vi "Update Plugin Metadata by Reference.vi"(8 "error in (no error)":errorcluster, 10 "plugin_metadata":T1, 11 "Metadata":refnum<vi>) -> (0 "error out":errorcluster)   [LabVIEW 2021, in "CIF_UI.lvclass"]
uses:
  CIF_UI.lvclass
  CIF_UI.lvclass/CIF_UI.ctl
  CIFPluginManager/CIFPluginManager/gRPC/CIF_Manager_client/RPC Messages/cif_manager_PluginMetadata.ctl
  CIFPluginManager/CIFPluginManager/gRPC/CIF_Manager_client/CIF_Manager_client.lvlib
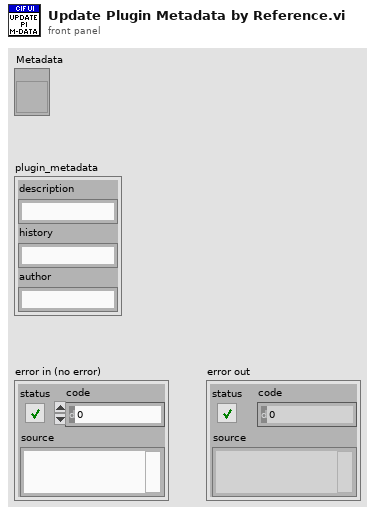
[diagram p1: front panel]
types:
  T1 = typedef "CIF_Manager_client.lvlib/cif_manager_PluginMetadata.ctl" = cluster{"description":string, "history":string, "author":string}
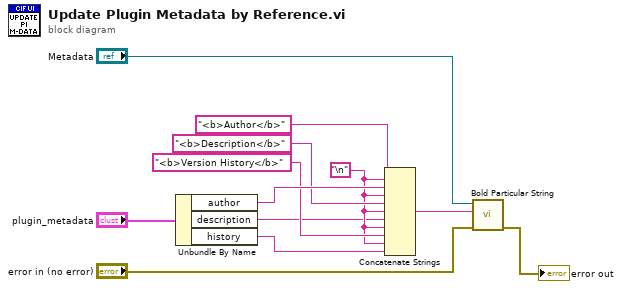
[diagram p0: block diagram]
diagram:
  w7 = "\n"
  n1 = Unbundle By Name("plugin_metadata") -> ("author"=w10:string, "description"=w6:string, "history"=w5:string)
  n2 = Concatenate Strings("<b>Author</b>" ("string"), w7, w10, w7, "<b>Description</b>" ("string"), w7, w6, w7, "<b>Version History</b>" ("string"), w7, w5) -> (w4:string)
  n3 = call <vilib>:"Bold Particular String.vi"("error in (no error)"="error in (no error)", "text to display"=w4, "string refnum"="Metadata") -> ("error out"=→"error out":errorcluster)  [unwired: 7 in, 1 out]
